vi "Configure Multi Eval Meas Limit SEM Additional Channel BW.vi"(0 "VISA resource name":refnum<visa-resource-name>, 1 "Bandwidth (5 MHz)":T1=5 items=["5 MHz"=5, "10 MHz"=10, "15 MHz"=15, "20 MHz"=20, "25 MHz"=25, "30 MHz"=30, "40 MHz"=40, "50 MHz"=50, "60 MHz"=60, "80 MHz"=80, "90 MHz"=90, "100 MHz"=100], 2 "Frequency Start (0Hz)":dbl format="%#.9p", 3 "Level (0.0)":dbl format="%^.3e", 5 "Instance (1)":T4=1, 7 "Area (1)":T3=1, 9 "Table (1)":T2=1, 11 "error in (no error)":errorcluster, 12 "Enable (Off)":bool, 13 "Frequency End (0Hz)":dbl format="%#.9p", 14 "RBW (30 kHz)":i32(ring) items=["30 kHz", "100 kHz", "1 MHz", "1 % of channel bandwidth", "2 % of channel bandwidth"]) -> (4 "VISA resource name out":refnum<visa-resource-name>, 15 "error out":errorcluster)   [LabVIEW 2020, in "Rohde&Schwarz CMWXP NR FR1 Measurement.lvlib"]
doc: "Defines additional requirements for the emission mask area number <area> (for NR SA). The activation state, the area borders, an upper limit and the resolution bandwidth must be specified.\nThe emission mask applies to the channel bandwidth <bw>. Several tables of additional requirements are available.\n\nAttribute:\nRSCMWXPNRFR1M_ATTR_MULTI_EVAL_MEAS_LIMIT_SEM_ADDITIONAL_CHANNEL_BW\n\nRemote-control command:\nCONFigure:NRSub:MEAS<i>:MEValuation:LIMit:SEMask:AREA<area>:ADDitional<table>:CBANdwidth<bw>"
uses:
  <instrlib>/Rohde&Schwarz CMWXP NR FR1 Measurement/Rohde&Schwarz CMWXP NR FR1 Measurement.lvlib
  <instrlib>/Rohde&Schwarz CMWXP NR FR1 Measurement/Private/_Instance.ctl
  <instrlib>/Rohde&Schwarz CMWXP NR FR1 Measurement/Private/_Area.ctl
  <instrlib>/Rohde&Schwarz CMWXP NR FR1 Measurement/Private/_Table.ctl
  <instrlib>/Rohde&Schwarz CMWXP NR FR1 Measurement/Private/_Bandwidth.ctl
  <instrlib>/Rohde&Schwarz CMWXP NR FR1 Measurement/Private/rsidr_core.llb/rsidr_core.lvlib
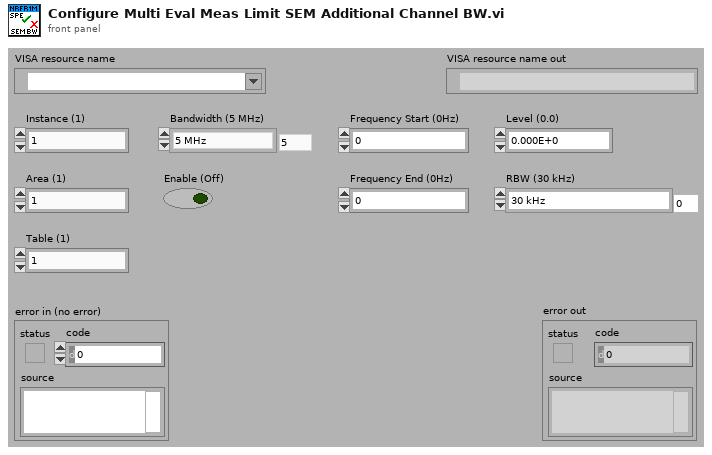
[diagram p1: front panel]
types:
  T1 = typedef "Rohde&Schwarz CMWXP NR FR1 Measurement.lvlib/_Bandwidth.ctl" = i32
  T2 = typedef "Rohde&Schwarz CMWXP NR FR1 Measurement.lvlib/_Table.ctl" = i32
  T3 = typedef "Rohde&Schwarz CMWXP NR FR1 Measurement.lvlib/_Area.ctl" = i32
  T4 = typedef "Rohde&Schwarz CMWXP NR FR1 Measurement.lvlib/_Instance.ctl" = i32
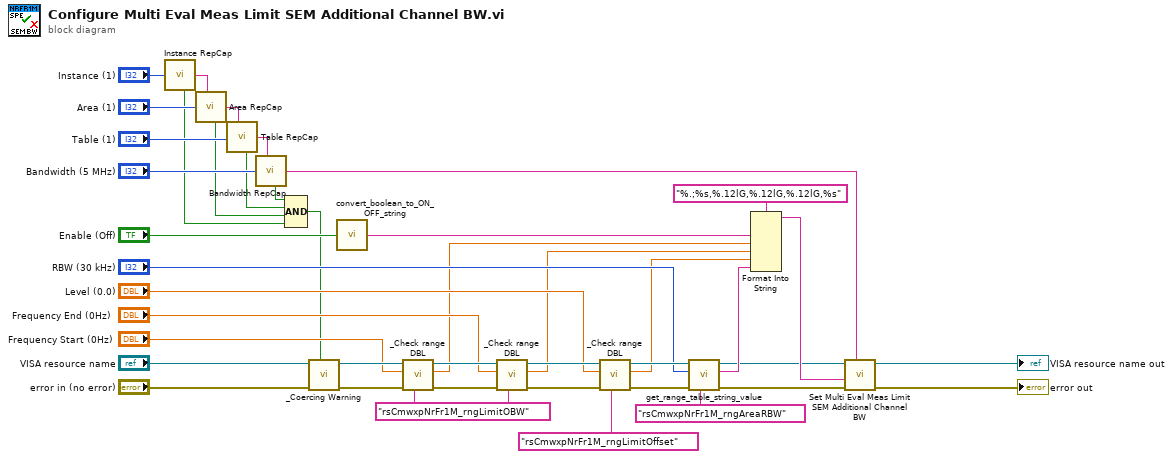
[diagram p0: block diagram]
diagram:
  w11 = "rsCmwxpNrFr1M_rngLimitOBW" ("Range Table Identifier")
  n1 = call <instrlib>:"Instance RepCap.vi"("Instance In"="Instance (1)") -> ("In Range?"=w2:bool, "RepCap Identifier Out"=w39:string)  [unwired: 1 in]
  n2 = call <instrlib>:"Area RepCap.vi"("SEM Area In"="Area (1)", "RepCap String In (\"\")"=w39) -> ("In Range?"=w3:bool, "RepCap Identifier Out"=w36:string)
  n3 = call <instrlib>:"Table RepCap.vi"("Table In"="Table (1)", "RepCap String In (\"\")"=w36) -> ("In Range?"=w4:bool, "RepCap Identifier Out"=w8:string)
  n4 = call <instrlib>:"Bandwidth RepCap.vi"("Bandwidth (5 MHz)"="Bandwidth (5 MHz)", "RepCap String In (\"\")"=w8) -> ("In Range?"=w5:bool, "RepCap Identifier Out"=w6:string)
  n5 = Compound Arithmetic op=AND(w5, w4, w3, w2) -> (w1:bool)
  n6 = call <instrlib>:"_Coercing Warning.vi"("In Range?"=w1, "error in (no error)"="error in (no error)", "VISA resource name"="VISA resource name") -> ("error out"=w30:errorcluster, "VISA resource name out"=w29:refnum<visa-resource-name>)  [unwired: 7 in]
  n7 = call <instrlib>:"convert_boolean_to_ON_OFF_string.vi"("boolean value in"="Enable (Off)") -> ("string value out"=w31:string)  [unwired: 4 in]
  n8 = call <instrlib>:"_Check range DBL.vi"("Range Table Identifier"=w11, "error in (no error)"=w30, "DBL Value In"="Frequency Start (0Hz)", "VISA resource name"=w29) -> ("error out"=w28:errorcluster, "DBL Value Out"=w18:dbl, "VISA resource name out"=w27:refnum<visa-resource-name>)  [unwired: 5 in]
  n9 = call <instrlib>:"_Check range DBL.vi"("Range Table Identifier"=w11, "error in (no error)"=w28, "DBL Value In"="Frequency End (0Hz)", "VISA resource name"=w27) -> ("error out"=w26:errorcluster, "DBL Value Out"=w17:dbl, "VISA resource name out"=w25:refnum<visa-resource-name>)  [unwired: 5 in]
  n10 = call <instrlib>:"_Check range DBL.vi"("Range Table Identifier"="rsCmwxpNrFr1M_rngLimitOffset", "error in (no error)"=w26, "DBL Value In"="Level (0.0)", "VISA resource name"=w25) -> ("error out"=w24:errorcluster, "DBL Value Out"=w16:dbl, "VISA resource name out"=w23:refnum<visa-resource-name>)  [unwired: 5 in]
  n11 = call <instrlib>:"get_range_table_string_value.vi"("Range Table ID in"="rsCmwxpNrFr1M_rngAreaRBW", "error in"=w24, "I32 input"="RBW (30 kHz)", "VISA resource name"=w23) -> ("error out"=w12:errorcluster, "String Value out"=w15:string, "VISA resource name out"=w13:refnum<visa-resource-name>)  [unwired: 5 in]
  n12 = Format Into String(format string="%.;%s,%.12lG,%.12lG,%.12lG,%s", w31, w18, w17, w16, w15) -> (resulting string=w14:string)  [unwired: 2 in, 1 out]
  n13 = call "Set Multi Eval Meas Limit SEM Additional Channel BW"("Repeated Capabilities"=w6, "error in (no error)"=w12, "Multi Eval Meas Limit SEM Additional Channel BW ()"=w14, "instrument handle"=w13) -> ("error out"=→"error out":errorcluster, "instrument handle out"=→"VISA resource name out":refnum<visa-resource-name>)  [unwired: 6 in]
